vi "Reflect Setting.vi"(7 "Depth":T1 items=["WRITE AREA", "RUNNING AREA", "SAVE AREA"], 8 "error in (no error)":errorcluster, 11 "Device ID (0)":i32) -> (0 "error out":errorcluster, 2 "Setting Error":u32 format="%.0x", 3 "Device ID out":i32)   [LabVIEW 2015, in "KEYENCE LJ-X8000A.lvlib"]
doc: "When the controller was instructed to reflect settings to the save area with this function,\nensure that you check the access status to the save area with the\n<B>Check Status of Saving to Save Area</B> VI before turning the power off."
uses:
  KEYENCE LJ-X8000A.lvlib
  Constants/Setting Depth.ctl
panel:
  # "(c) 2019 KEYENCE CORPORATION.  ALL RIGHTS RESERVED."
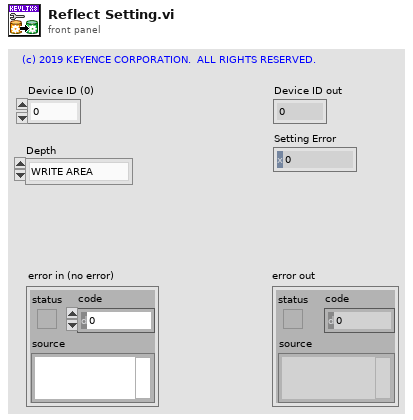
[diagram p1: front panel]
types:
  T1 = typedef "KEYENCE LJ-X8000A.lvlib/Setting Depth.ctl" = u8
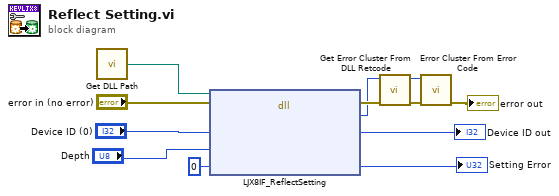
[diagram p0: block diagram]
diagram:
  n1 = call "Get DLL Path.vi"() -> ("DLL Path"=w8:path)  [unwired: 3 in]
  n2 = dll-call lib="C:/Program Files (x86)/National Instruments/LabVIEW 2018/instr.lib/KEYENCE LJ-X8000/LJX8_IF.*" fn="LJX8IF_ReflectSetting"(path in=w8, error in="error in (no error)", "lDeviceId"="Device ID (0)", "byDepth"="Depth", "pdwError"=u32 0) -> (error out=w6:errorcluster, "lRetCode"=w5:i32, "lDeviceId"=→"Device ID out":i32, "pdwError"=→"Setting Error":u32)  [unwired: 2 in, 1 out]
  n3 = call "Get Error Cluster From DLL Retcode.vi"("error in (no error)"=w6, "DLL Return Code"=w5) -> ("error out"=w7:errorcluster, "VI Error Code"=w1:i32)  [unwired: 8 in]
  n4 = call <vilib>:"Error Cluster From Error Code.vi"("error in (no error)"=w7, "error code (0)"=w1) -> ("error out"=→"error out":errorcluster)  [unwired: 7 in]
